vi "UseDeviceKey.vi"() -> ()   [LabVIEW 2009]
uses:
  C:/Samples/LabVIEW/UseDeviceKey/LabVIEW 2009/UsbDllWrap.dll
panel:
  out "Output:":string
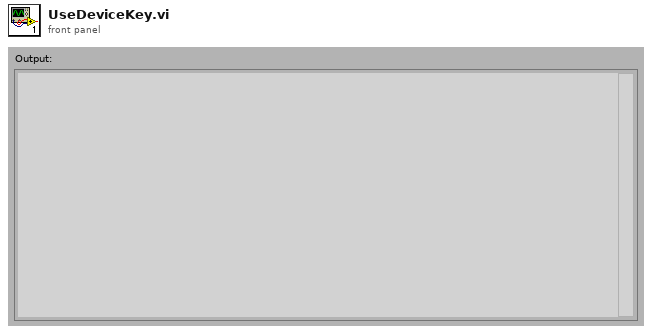
[diagram p1: front panel]
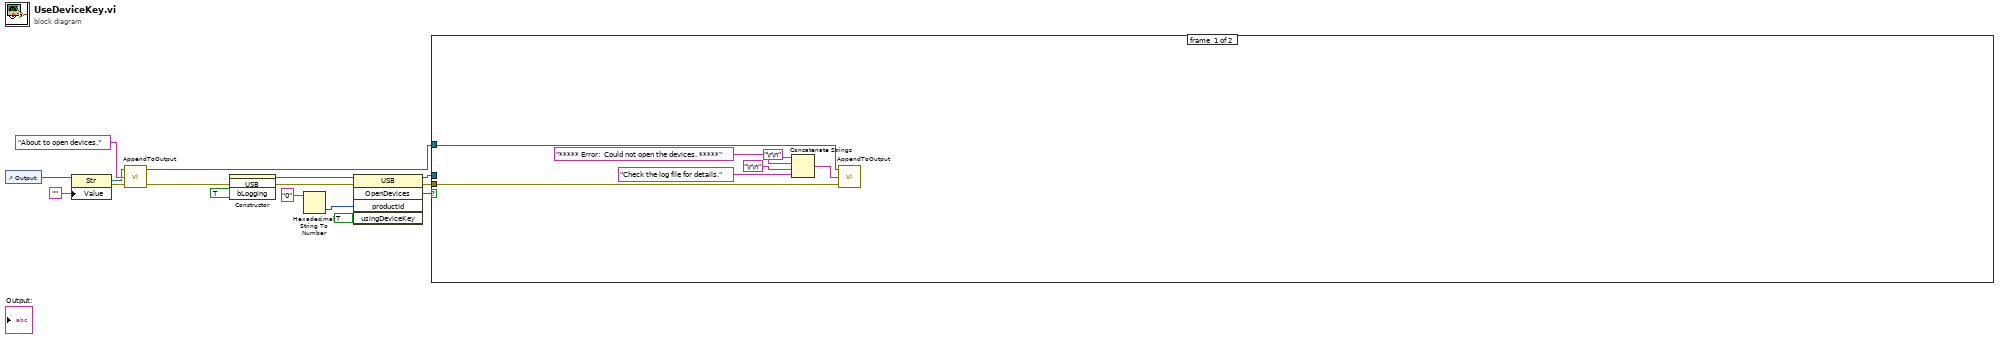
[diagram p0: block diagram]
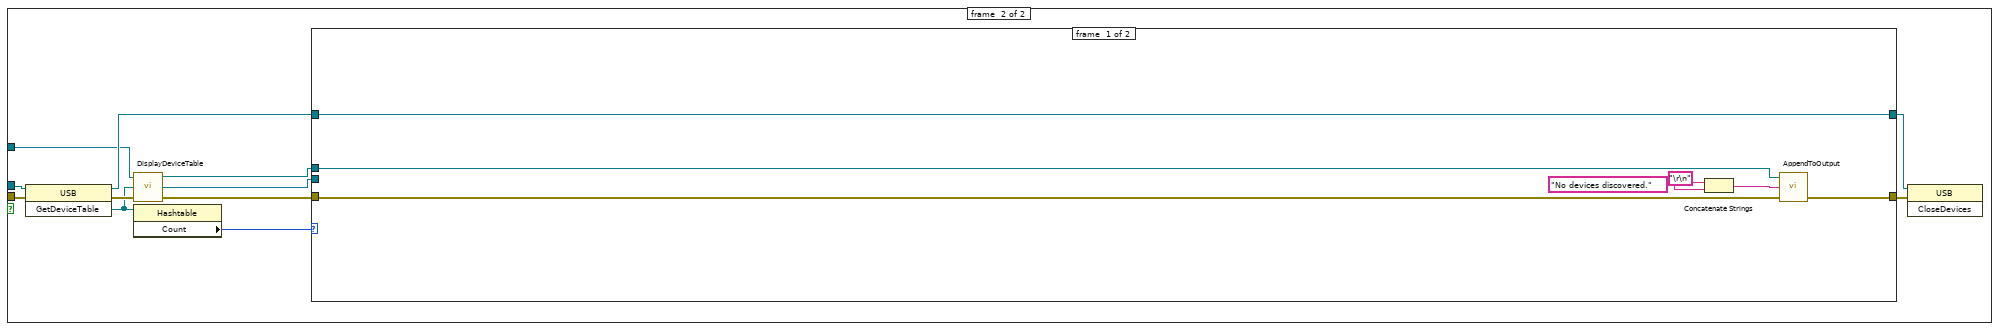
[diagram p2: hidden frame]
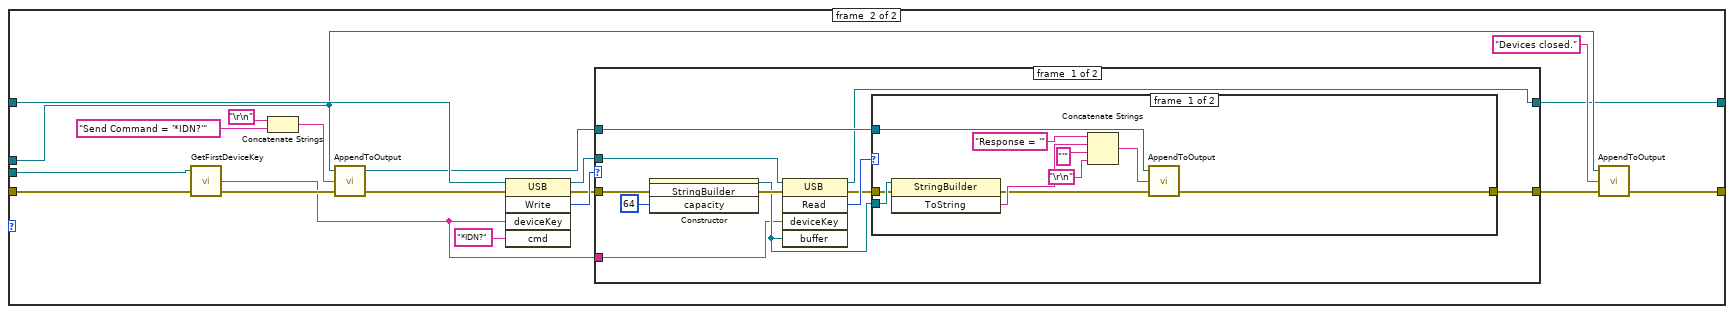
[diagram p3: hidden frame]
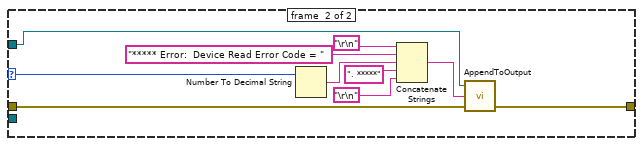
[diagram p4: hidden frame]
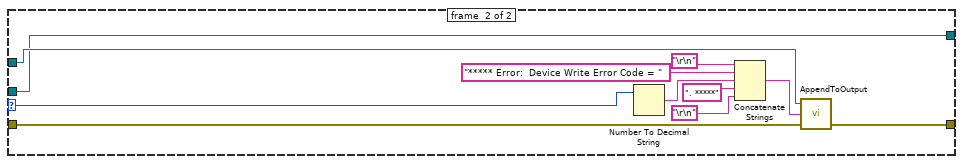
[diagram p5: hidden frame]
diagram:
  n1 = control-ref of="Output:"() -> (w7:refnum<vi>)
  n2 = property class="Str"(reference=w7, "Value"="") -> (reference out=w4:refnum<vi>, error out=w5:errorcluster)  [unwired: 1 in]
  n3 = call "AppendToOutput.vi"("error in"=w5, "Input String"="About to open devices.", "Output Refnum In"=w4) -> ("error out"=w14:errorcluster, "Output Refnum Out"=w11:refnum<vi>)  [unwired: 1 in]
  n4 = constructor class="USB"(error in=w14, "bLogging"=TRUE) -> (reference out=w13:refnum<k24>, error out=w10:errorcluster)  [unwired: 2 in, 2 out]
  n5 = Hexadecimal String To Number(string="0") -> (number=w2:u32)  [unwired: 2 in, 1 out]
  n6 = invoke class="USB" method="OpenDevices"(reference=w13, error in=w10, "productId"=w2, "usingDeviceKey"=TRUE) -> (reference out=w8:refnum<k24>, error out=w9:errorcluster, "OpenDevices"=w12:bool)  [unwired: 1 in, 2 out]
  n7 = case shown="True" w12 {
    tunnel: w11 -> [w23 w31]
    tunnel: w9 -> [w22 w34]
    tunnel: w8 -> [_ w35]
    frame #0 {
      n8 = Concatenate Strings("\r\n", "***** Error:  Could not open the devices. *****", "\r\n", "Check the log file for details.") -> (w18:string)
      n9 = call "AppendToOutput.vi"("error in"=w22, "Input String"=w18, "Output Refnum In"=w23) -> ()  [unwired: 1 in, 2 out]
    }
    frame #1 {
      n10 = invoke class="USB" method="GetDeviceTable"(reference=w35, error in=w34) -> (reference out=w33:refnum<k24>, error out=w30:errorcluster, "GetDeviceTable"=w26:refnum<k24>)  [unwired: 1 in]
      n11 = call "DisplayDeviceTable.vi"("error in (no error)"=w30, "Device Table In"=w26, "Output Refnum In"=w31) -> ("error out"=w32:errorcluster, "Device Table Out"=w28:refnum<k24>, "Output Refnum Out"=w29:refnum<vi>)
      n12 = property class="Hashtable"(reference=w26) -> ("Count"=w27:i32)  [unwired: 1 in, 2 out]
      n13 = case shown="1, Default" w27 {
        tunnel: w33 -> [w36 w57]
        tunnel: w32 -> [w39 w47]
        tunnel: w29 -> [w38 w46]
        tunnel: w28 -> [_ w45]
        tunnel: [w37 w44] -> w25
        tunnel: [w36 w43] -> w24
        frame #0 {
          n14 = Concatenate Strings("\r\n", "No devices discovered." ("string")) -> (w40:string)
          n15 = call "AppendToOutput.vi"("error in"=w39, "Input String"=w40, "Output Refnum In"=w38) -> ("error out"=w37:errorcluster)  [unwired: 1 in, 1 out]
        }
        frame #1 {
          n16 = call "GetFirstDeviceKey.vi"("error in (no error)"=w47, "Device Table In"=w45) -> ("error out"=w55:errorcluster, "Device Key"=w48:string)  [unwired: 1 in, 1 out]
          n17 = Concatenate Strings("\r\n", "Send Command = '*IDN?'") -> (w59:string)
          n18 = call "AppendToOutput.vi"("error in"=w55, "Input String"=w59, "Output Refnum In"=w46) -> ("error out"=w56:errorcluster, "Output Refnum Out"=w51:refnum<vi>)  [unwired: 1 in]
          n19 = invoke class="USB" method="Write"(reference=w57, error in=w56, "deviceKey"=w48, "cmd"="*IDN?") -> (reference out=w53:refnum<k24>, error out=w52:errorcluster, "Write"=w54:i32)  [unwired: 1 in, 2 out]
          n20 = case shown="0" w54 {
            selector: w54 -> [_ w98]
            tunnel: w53 -> [w72 w93]
            tunnel: w52 -> [w69 w96]
            tunnel: [w65 w95] -> w49
            tunnel: w51 -> [w64 w94]
            tunnel: w48 -> [w63 _]
            tunnel: [w62 w93] -> w43
            frame #0 {
              n21 = constructor class="StringBuilder"(error in=w69, "capacity"=64) -> (reference out=w67:refnum<k24>, error out=w70:errorcluster)  [unwired: 2 in, 2 out]
              n22 = invoke class="USB" method="Read"(reference=w72, error in=w70, "deviceKey"=w63, "buffer"=w67) -> (reference out=w62:refnum<k24>, error out=w66:errorcluster, "Read"=w68:i32)  [unwired: 1 in, 2 out]
              n23 = case shown="0" w68 {
                selector: w68 -> [_ w87]
                tunnel: w67 -> [w82 _]
                tunnel: w66 -> [w81 w84]
                tunnel: [w74 w83] -> w65
                tunnel: w64 -> [w73 w85]
                frame #0 {
                  n24 = invoke class="StringBuilder" method="ToString"(reference=w82, error in=w81) -> (error out=w75:errorcluster, "ToString"=w78:string)  [unwired: 1 in, 1 out]
                  n25 = Concatenate Strings("Response = '", w78, "'", "\r\n") -> (w76:string)
                  n26 = call "AppendToOutput.vi"("error in"=w75, "Input String"=w76, "Output Refnum In"=w73) -> ("error out"=w74:errorcluster)  [unwired: 1 in, 1 out]
                }
                frame #1 {
                  n27 = Number To Decimal String(number=w87) -> (decimal integer string=w92:string)  [unwired: 1 in]
                  n28 = Concatenate Strings("\r\n", "***** Error:  Device Read Error Code = ", w92, ". *****", "\r\n") -> (w86:string)
                  n29 = call "AppendToOutput.vi"("error in"=w84, "Input String"=w86, "Output Refnum In"=w85) -> ("error out"=w83:errorcluster)  [unwired: 1 in, 1 out]
                }
              }
            }
            frame #1 {
              n30 = Number To Decimal String(number=w98) -> (decimal integer string=w99:string)  [unwired: 1 in]
              n31 = Concatenate Strings("\r\n", "***** Error:  Device Write Error Code = ", w99, ". *****", "\r\n") -> (w97:string)
              n32 = call "AppendToOutput.vi"("error in"=w96, "Input String"=w97, "Output Refnum In"=w94) -> ("error out"=w95:errorcluster)  [unwired: 1 in, 1 out]
            }
          }
          n33 = call "AppendToOutput.vi"("error in"=w49, "Input String"="Devices closed." ("string"), "Output Refnum In"=w46) -> ("error out"=w44:errorcluster)  [unwired: 1 in, 1 out]
        }
      }
      n34 = invoke class="USB" method="CloseDevices"(reference=w24, error in=w25) -> ()  [unwired: 1 in, 3 out]
    }
  }
